vi "AIT 1553 BM HWIn Loop.vi"(11 "RT Data":T1 {"Acyclic Frame Refs" format="%.0x"; "Label Transfer Config"."Block Data Refs"."Data Reference" format="%.0x"; "Status Config"."HWOut Dur Ref" format="%.0x"; "Status Config"."HWIn Dur Ref" format="%.0x"; "Status Config"."HWOut Count Ref" format="%.0x"; "Status Config"."HWIn Count Ref" format="%.0x"; "Status Config"."Error Data Ref" format="%.0x"; "HWOutput Channels"."Message Settings"."Driver Data"."First Word" min=8 max=31; "HWOutput Channels"."Message Settings"."Driver Data"."Num Bits" min=1 max=32; "HWOutput Channels"."Message Settings"."Driver Data"."Start Bit" min=8 max=31; "HWOutput Channels"."Message Settings"."Block Data Refs"."Data Reference" format="%.0x"; "HWInput Channels"."Message Settings"."Driver Data"."First Word" min=8 max=31; "HWInput Channels"."Message Settings"."Driver Data"."Num Bits" min=1 max=32; "HWInput Channels"."Message Settings"."Driver Data"."Start Bit" min=8 max=31; "HWInput Channels"."Message Settings"."Block Data Refs"."Data Reference" format="%.0x"}) -> ()   [LabVIEW 2013, in "AIT 1553 Custom Device.lvlib"]
uses:
  AIT 1553 Custom Device.lvlib
  RT Controls/AIT 1553  - RT Data.ctl
  RT Controls/AIT 1553 - RT HW Channel.ctl
  RT Controls/AIT 1553 - Bus Section.ctl
  RT Controls/AIT 1553 - RT Message Settings.ctl
  <vilib>/NI Veristand/Custom Device API/Block Data Reference.ctl
  <vilib>/NI Veristand/Custom Device API/Data Reference.ctl
  RT Controls/AIT 1553 - Driver Data.ctl
  Controls and Global/Start Bit.ctl
  Controls and Global/Number of Bits.ctl
  RT Controls/AIT 1553 - Board Config Info.ctl
  RT Controls/AIT 1553 - Hardware Type.ctl
  RT Controls/Error Qs.ctl
  RT Controls/Status Channels Config.ctl
  RT Controls/FIFO.ctl
  RT Controls/Label Transfer Config.ctl
  <vilib>/NI Veristand/Custom Device API/Custom Device Item Ref.ctl
  <vilib>/Platform/TimedLoop/XDataNode/timing_clust.ctl
  <vilib>/Platform/TimedLoop/XDataNode/nitl_modes.ctl
  <vilib>/Platform/TimedLoop/XDataNode/wakeup.ctl
  RT Controls/ReadWrite Selector.ctl
  <vilib>/Platform/TimedLoop/XDataNode/XDataNode.xnode
  <vilib>/Platform/TimedLoop/XDataNode/XDNodeRunTimeDep.lvlib
  <vilib>/NI Veristand/Custom Device API/Custom Device API.lvlib
panel:
  in  "stop":bool
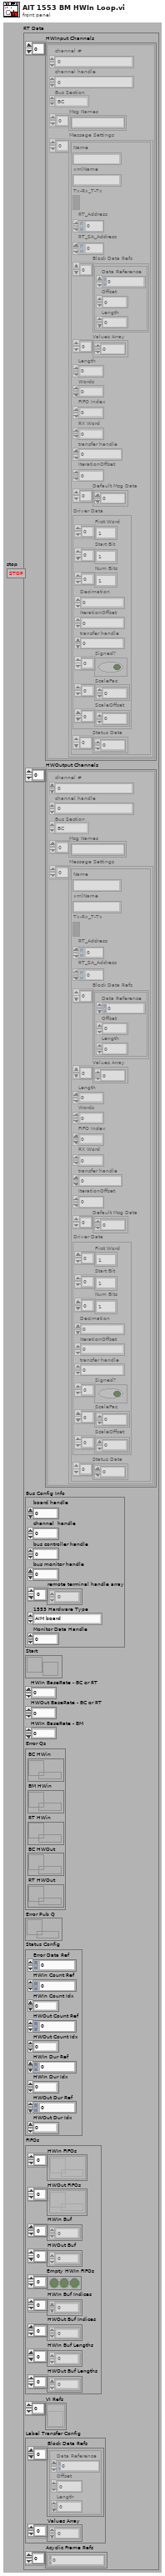
[diagram p1: front panel]
types:
  T1 = typedef "AIT 1553 Custom Device.lvlib/AIT 1553  - RT Data.ctl" = cluster{"HWInput Channels":T2[], "HWOutput Channels":T2[], "Bus Config Info":T10, "Start":refnum<notifier>, "HWIn BaseRate - BC or RT":i64, "HWOut BaseRate - BC or RT":i64, "HWIn BaseRate - BM":i64, "Error Qs":T12, "Error Pub Q":refnum<queue>, "Status Config":T13, "FIFOs":T14, "VI Refs":refnum<vi>[], "Label Transfer Config":T15, "Acyclic Frame Refs":T16[]}
  T2 = typedef "AIT 1553 Custom Device.lvlib/AIT 1553 - RT HW Channel.ctl" = cluster{"channel #":u16, "channel handle":u32, "Bus Section":T3, "Msg Names":string[], "Message Settings":T4[]}
  T3 = typedef "AIT 1553 Custom Device.lvlib/AIT 1553 - Bus Section.ctl" = enum16{"BC", "BM", "RT"}
  T4 = typedef "AIT 1553 Custom Device.lvlib/AIT 1553 - RT Message Settings.ctl" = cluster{"Name":string, "xmlName":string, "Tx-Rx_T-Tx":bool, "RT_Address":u8, "RT_SA_Address":u8, "Block Data Refs":T5[], "Values Array":dbl[], "Length":i32, "Words":i32, "FIFO Index":i32, "RX Word":u32, "transfer handle":u32, "IterationOffset":i32, "Default Msg Data":u16[], "Driver Data":T7, "Status Data":u32[]}
  T5 = typedef "Custom Device API.lvlib/Block Data Reference.ctl" = cluster{"Data Reference":T6, "Offset":i32, "Length":i32}
  T6 = typedef "Custom Device API.lvlib/Data Reference.ctl" = i32
  T7 = typedef "AIT 1553 Custom Device.lvlib/AIT 1553 - Driver Data.ctl" = cluster{"First Word":T8[], "Start Bit":T8[], "Num Bits":T9[], "Decimation":i32, "IterationOffset":i32, "transfer handle":u32, "Signed?":bool[], "ScaleFac":dbl[], "ScaleOffset":dbl[]}
  T8 = typedef "AIT 1553 Custom Device.lvlib/Start Bit.ctl" = i32
  T9 = typedef "AIT 1553 Custom Device.lvlib/Number of Bits.ctl" = i32
  T10 = typedef "AIT 1553 Custom Device.lvlib/AIT 1553 - Board Config Info.ctl" = cluster{"board handle":u32, "channel  handle":u32, "bus controller handle":u32, "bus monitor handle":u32, "remote terminal handle array":u32[], "1553 Hardware Type":T11, "Monitor Data Handle":u32}
  T11 = typedef "AIT 1553 Custom Device.lvlib/AIT 1553 - Hardware Type.ctl" = enum16{"AIM board", "AIT Board"}
  T12 = typedef "AIT 1553 Custom Device.lvlib/Error Qs.ctl" = cluster{"BC HWin":refnum<queue>, "BM HWin":refnum<queue>, "RT HWin":refnum<queue>, "BC HWOut":refnum<queue>, "RT HWOut":refnum<queue>}
  T13 = typedef "AIT 1553 Custom Device.lvlib/Status Channels Config.ctl" = cluster{"Error Data Ref":T6, "HWIn Count Ref":T6, "HWIn Count Idx":i32, "HWOut Count Ref":T6, "HWOut Count Idx":i32, "HWIn Dur Ref":T6, "HWIn Dur Idx":i32, "HWOut Dur Ref":T6, "HWOut Dur Idx":i32}
  T14 = typedef "AIT 1553 Custom Device.lvlib/FIFO.ctl" = cluster{"HWIn FIFOs":refnum<k33>[], "HWOut FIFOs":refnum<k33>[], "HWIn Buf":dbl[], "HWOut Buf":dbl[], "Empty HWIn FIFOs":bool[], "HWIn Buf Indices":i32[], "HWOut Buf Indices":i32[], "HWIn Buf Lengths":i32[], "HWOut Buf Lengths":i32[]}
  T15 = typedef "AIT 1553 Custom Device.lvlib/Label Transfer Config.ctl" = cluster{"Block Data Refs":T5[], "Values Array":dbl[]}
  T16 = typedef "Custom Device API.lvlib/Custom Device Item Ref.ctl" = u64
  T17 = typedef "AIT 1553 Custom Device.lvlib/ReadWrite Selector.ctl" = enum16{"Inline Read", "Inline Write", "Async HWIn", "Async HWOut"}
  T18 = typedef "XDNodeRunTimeDep.lvlib/timing_clust.ctl" = cluster{"Expected End [f-1]":u64, "Actual End [f-1]":u64, "Finished Late? [f-1]":bool, "Expected End [i-1]":u64, "Actual End [i-1]":u64, "Finished Late? [i-1]":bool, "Expected Start [i]":u64, "Actual Start [i]":u64, "Expected Start [f]":u64, "Actual Start [f]":u64, "Source Name":string, "Structure Name":string, "Period":i64, "Deadline":i64, "Offset":i64, "Start":i64, "Priority":i32, "Timeout":i32, "Mode":T19, "Wakeup Reason":T20, "Error":errorcluster, "Source Type":string, "Secondary Source Type":string, "Global End Time":u64, "Global Start Time":u64, "Frame Duration":u64, "Iteration Duration":u64, "Assigned CPU":i32, "I/O Scan Engine Mode":u32}
  T19 = typedef "XDNodeRunTimeDep.lvlib/nitl_modes.ctl" = enum32{"No Change", "Process missed periods, maintain original phase", "Discard missed periods, maintain original phase", "Process missed periods, ignore original phase", "Discard missed periods, ignore original phase"}
  T20 = typedef "XDNodeRunTimeDep.lvlib/wakeup.ctl" = enum32{"Normal", "Aborted", "Asynchronous wakeup", "Timing source error", "Timed loop error", "Timeout"}
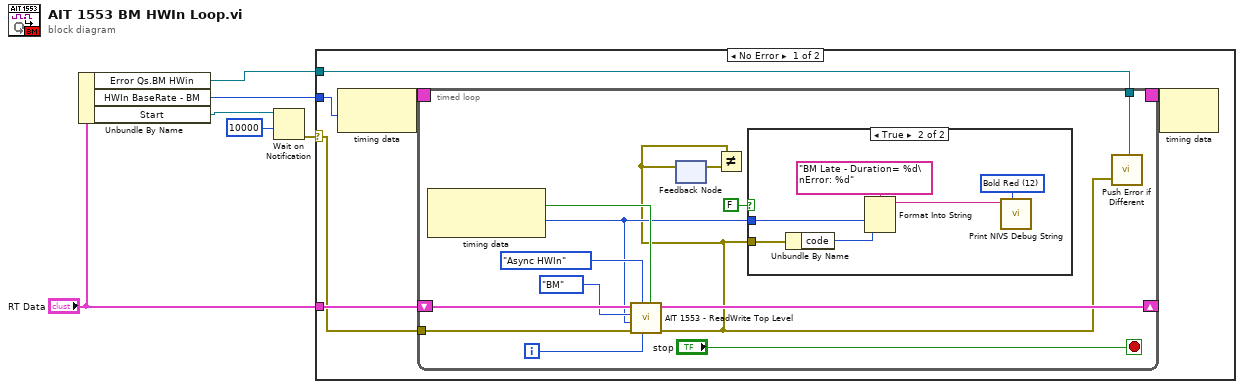
[diagram p0: block diagram]
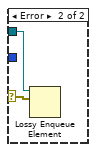
[diagram p3: hidden frame]
diagram:
  n1 = Unbundle By Name("RT Data") -> ("Error Qs.BM HWin"=w1:refnum<queue>, "HWIn BaseRate - BM"=w6:i64, "Start"=w5:refnum<notifier>)
  n2 = Wait on Notification(notifier=w5, timeout in ms (-1)=10000) -> (error out=w4:errorcluster)  [unwired: 2 in, 3 out]
  n3 = case shown="No Error" w4 {
    selector: w4 -> [w7 w41]
    tunnel: w6 -> [w10 _]
    tunnel: "RT Data" -> [w9 _]
    tunnel: w1 -> [w8 w40]
    frame No Error {
      n4 = node-c288(w10) -> (w12:T18)
      n5 = timed-loop {
        timing: w12 -> [_]
        timing-out: [_] -> w11
        shift-right: [w23] -> _
        shift-left: w9 -> [w24]
        tunnel: w8 -> [w21]
        tunnel: w7 -> [w20]
        i -> [w16]
        stop <- "stop" stop-if-true
        n6 = node-c288() -> (w18:bool, w17:i64)  [unwired: 1 in]
        n7 = call "AIT 1553 - ReadWrite Top Level.vi"("Late?"=w18, "Iteration"=w16, "Mode"=ReadWrite_Selector."Async HWIn", "error in (no error)"=w20, "Iteration Duration"=w17, "Bus Section"=AIT_1553_-_Bus_Section."BM", "RT Data in"=w24) -> ("error out"=w14:errorcluster, "RT Data out"=w23:T1)  [unwired: 3 in]
        n8 = feedback #1() -> (w15:errorcluster)  [unwired: 1 in]
        n9 = feedback-in #1(w14) -> ()
        n10 = Not Equal?(x=w14, y=w15) -> ()  [unwired: 1 out]
        n11 = case shown="True" FALSE {
          tunnel: w17 -> [_ w29]
          tunnel: w14 -> [_ w27]
          frame False {
          }
          frame True {
            w31 = u16 12 items=["Plain White"=7, "Bold White"=15, "Bold Blue"=9, "Bold Green"=10, "Bold Red"=12] ("Color (Plain White)")
            n12 = Unbundle By Name(w27) -> ("code"=w26:i32)
            n13 = Format Into String(format string="BM Late - Duration= %d\nError: %d", w29, w26) -> (resulting string=w30:string)  [unwired: 2 in, 1 out]
            n14 = call "Print NIVS Debug String.vi"("Color (Plain White)"=w31, "Debug String"=w30) -> ()  [unwired: 8 in, 1 out]
          }
        }
        n15 = call "Push Error if Different.vi"("error in"=w14, "Error Q"=w21) -> ()  [unwired: 1 in]
      }
      n16 = node-c288(w11) -> ()  [unwired: 1 out]
    }
    frame Error {
      n17 = Lossy Enqueue Element(queue=w40, element=w41) -> ()  [unwired: 1 in, 4 out]
    }
  }
